vi "Write Log File Path.vi"(8 "error in (no error)":errorcluster, 10 "Log File Path":path, 11 "Abstract Log Consumer in":refnum<class "Abstract Log Consumer.lvclass">) -> (0 "error out":errorcluster, 3 "Abstract Log Consumer out":refnum<class "Abstract Log Consumer.lvclass">)   [LabVIEW 2020, in "Messaging.lvlib" / "Abstract Log Consumer.lvclass"]
uses:
  Abstract Log Consumer.lvclass
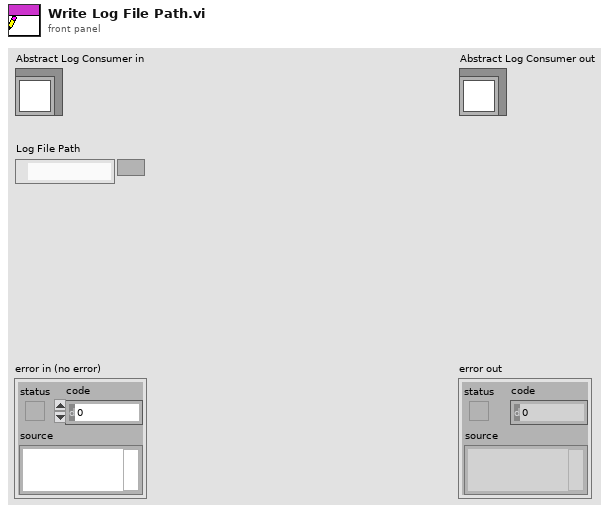
[diagram p1: front panel]
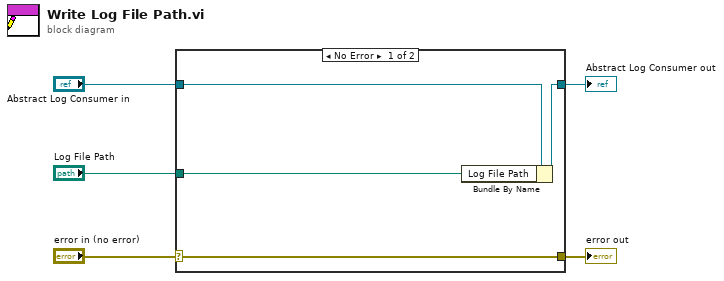
[diagram p0: block diagram]
diagram:
  n1 = case shown="No Error" "error in (no error)" {
    selector: "error in (no error)" -> [w9 w10]
    tunnel: [w9 w10] -> w4
    tunnel: [w7 w11] -> w2
    tunnel: "Abstract Log Consumer in" -> [w8 w11]
    tunnel: "Log File Path" -> [w6 _]
    frame No Error {
      n2 = Bundle By Name(cluster=w8, "Log File Path"=w6) -> (w7:refnum<class "Abstract Log Consumer.lvclass">)
    }
    frame Error {
    }
  }
  "error out" <- w4
  "Abstract Log Consumer out" <- w2
